vi "Instantiate with Reference.vi"(5 "VI Refnum":refnum<vi>, 11 "error in (no error)":errorcluster) -> (4 "Document.lvclass":refnum<class "Document.lvclass">, 15 "error out":errorcluster)   [LabVIEW 2016, in "LV RT.lvclass"]
uses:
  LV RT.lvclass
  Document.lvclass
  D:/MDI Project/source code/Document/Document.lvclass
  D:/MDI Project/source code/Document/Child Classes/LV Doc/LV Doc.lvclass
  LV Doc.lvclass/LV Doc.ctl
  LV Doc.lvclass
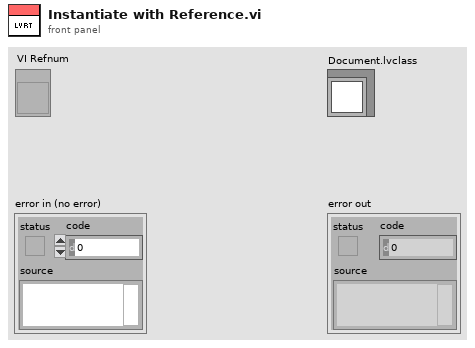
[diagram p1: front panel]
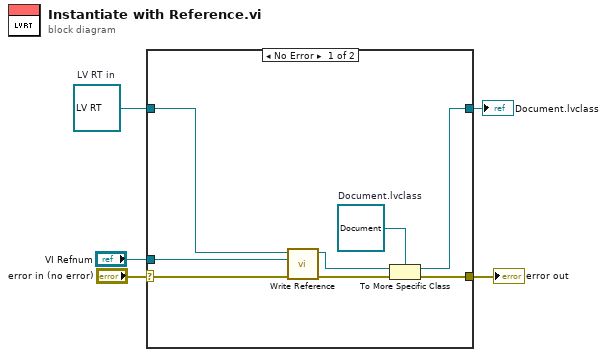
[diagram p0: block diagram]
diagram:
  w3 = refnum<class "LV RT.lvclass"> refnum  # LV RT in
  n1 = case shown="No Error" "error in (no error)" {
    selector: "error in (no error)" -> [w12 w15]
    tunnel: [w11 w15] -> w4
    tunnel: [w9 w14] -> w1
    tunnel: w3 -> [w10 w14]
    tunnel: "VI Refnum" -> [w6 _]
    frame No Error {
      w13 = refnum<class "Document.lvclass"> refnum  # Document.lvclass
      n2 = call "Write Reference.vi"("error in (no error)"=w12, "Reference"=w6, "LV Doc in"=w10) -> ("error out"=w8:errorcluster, "LV Doc out"=w7:refnum<class "LV RT.lvclass">)  [unwired: 7 in]
      n3 = To More Specific Class(target class=w13, reference=w7, error in=w8) -> (specific class reference=w9:refnum<class "Document.lvclass">, error out=w11:errorcluster)
    }
    frame Error {
    }
  }
  "error out" <- w4
  "Document.lvclass" <- w1
